vi "LEO PROVA MINCHIATA RT.vi"() -> ()   [LabVIEW 2014]
uses:
  <vilib>/FPGAPlugInAG/sbRIO-9636/niLvFpga_Open_sbRIO-9636.vi
  <vilib>/rvi/interface/common/dynamic/niFpgaDynamicAddResources.vi
  <vilib>/Utility/error.llb/Error Cluster From Error Code.vi
  <vilib>/rvi/errors/niLvFpgaAdjustHostInterfaceError.vi
  <vilib>/rvi/interface/common/niFpgaWaitOnOcc.vi
  <vilib>/FPGAPlugInAG/Dynamic/niLvFpga_Run_Dynamic.vi
  <vilib>/FPGAPlugInAG/Dynamic/niLvFpga_Abort_Dynamic.vi
  <vilib>/FPGAPlugInAG/Dynamic/niLvFpga_Close_Dynamic.vi
  <vilib>/rvi/interface/nirviOpenFPGA/nirviOpenFPGA.xnode
  FPGA Bitfiles/LaserDistanceSen_FPGATarget_LEOPROVAMINCHIAT_2r7d0oepUXA.lvbitx
  FPGA Target/Test VIs/LEO PROVA MINCHIATA.vi
  <vilib>/rvi/interface/nirviReadWriteControl/nirviReadWriteControl.xnode
  <vilib>/rvi/interface/nirviMethod/nirviMethod.xnode
  <vilib>/rvi/interface/nirviCloseFPGA/nirviCloseFPGA.xnode
  <vilib>/FPGAPlugInAG/Dynamic/niLvFpga_ConfigureFifo_Dynamic.vi
  <vilib>/rvi/errors/niLvFpgaMergeErrorWithErrorCode.vi
  <vilib>/FPGAPlugInAG/Dynamic/niLvFpga_StartFifo_Dynamic.vi
  <vilib>/rvi/interface/Simulation/niFpgaSimulationCallBeginRW.vi
  <vilib>/FPGAPlugInAG/Dynamic/niLvFpga_ReadFifo_Dynamic.vi
  NiFpgaLv.dll
panel:
  out "FFT (freq)":waveform(dbl)(graph)
  out "Signal (t)":waveform(dbl)(graph)
  in  "Snapshot":bool
  in  "Windowing":T1(ring)
  in  "first bin":i32=10
  in  "last bin":i32=255
  in  "lower limit 2":u32(slide)=677 scale=625.0..737.0
  in  "lower limit 1":u32(slide)=59 scale=0.0..112.0
  out "Detected Frequency Tone - (Hz)":dbl
  in  "stop":bool
  out "Max Bin":i32
  out "Max Amp":dbl format="%.2f"
  out "Prev Bin":i32
  out "Next Bin":i32
  out "Prev Amp":dbl format="%.2f"
  out "Next Amp":dbl format="%.2f"
  out "Interpolated Bin":dbl
  in  "Interpolation Method":T2(ring)=enum."Jain"
  # "WARNING:\nOnce pressed wait untill the end of operation"
  # "ONLINE parameter"
  # "OFFLINE parameters"
  # "Max Detection FFT bin range"
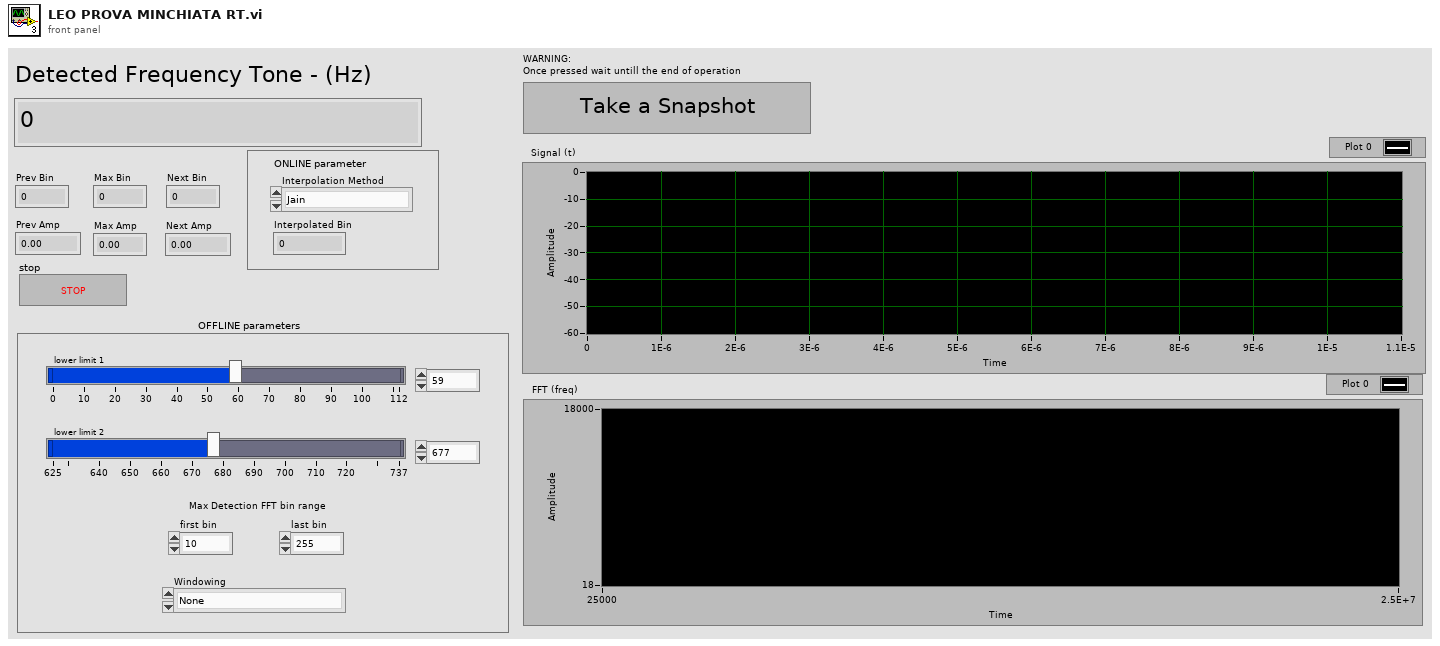
[diagram p1: front panel]
types:
  T1 = enum16{"None", "Hanning", "Hamming", "Blackman", "Blackman-Harris"}
  T2 = enum16{"Quadratic", "McLeodd", "Barycentric", "Jain"}
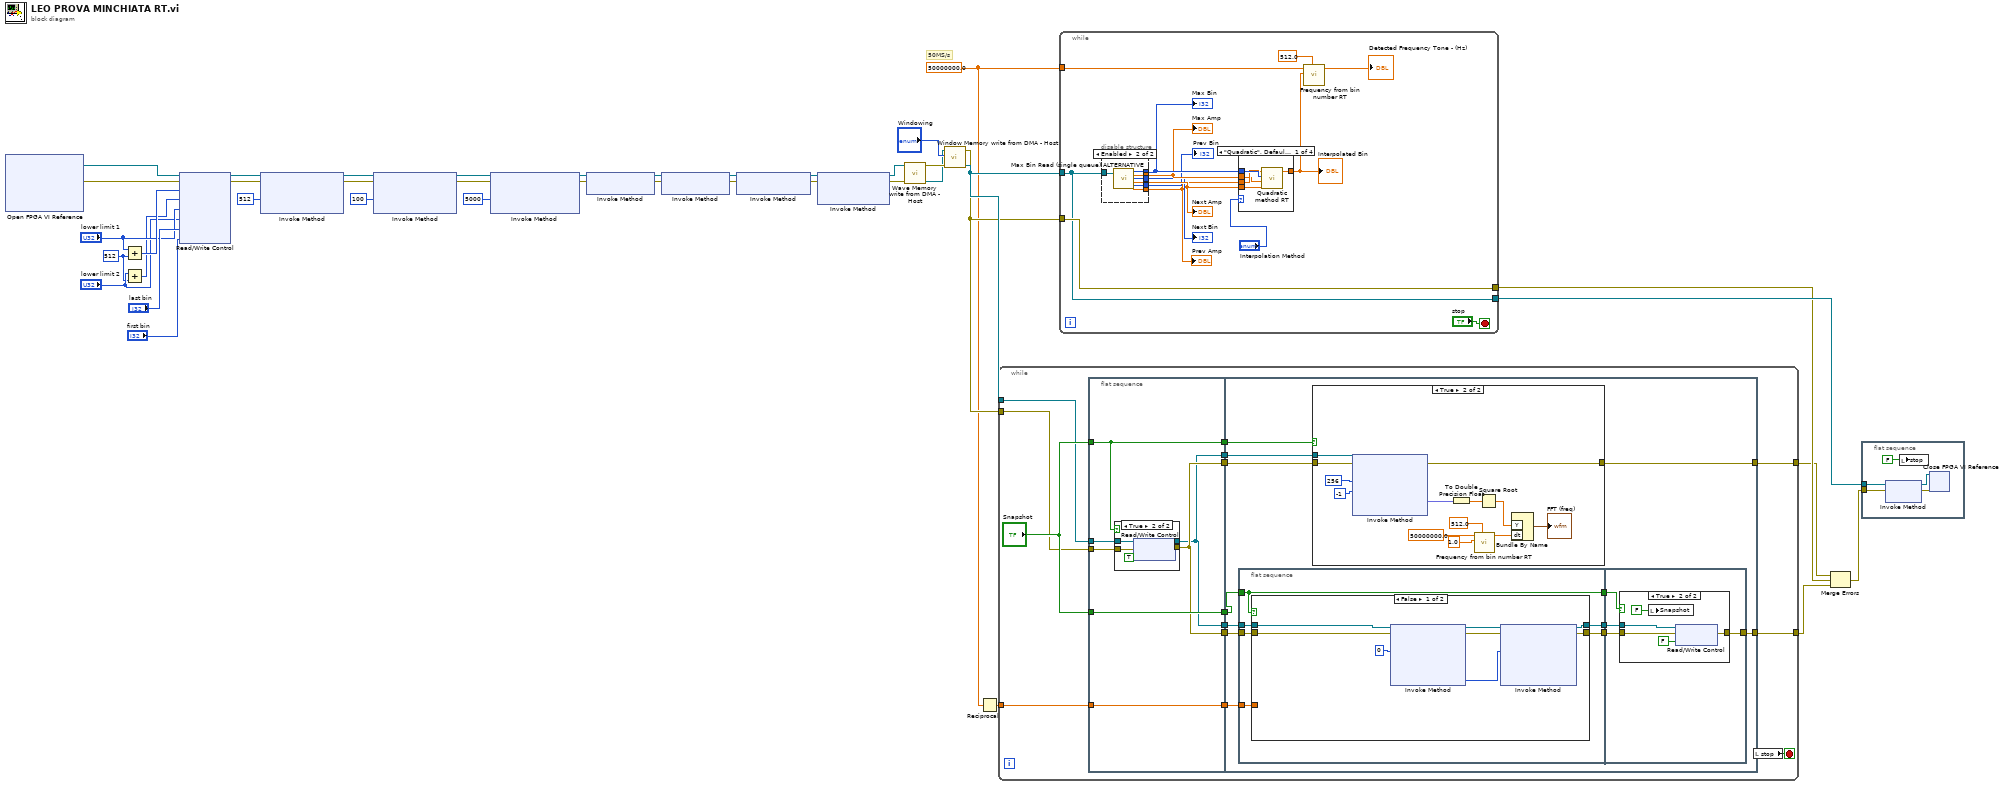
[diagram p0: block diagram]
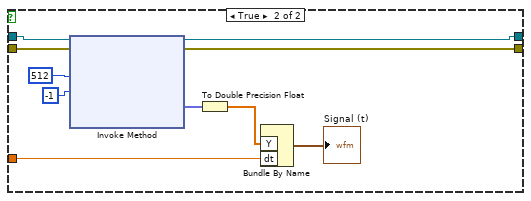
[diagram p3: hidden frame]
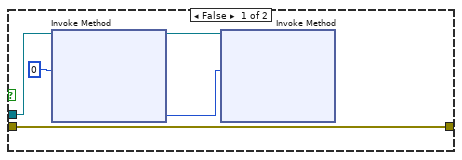
[diagram p5: hidden frame]
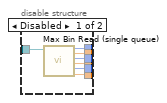
[diagram p6: hidden frame]
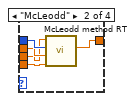
[diagram p7: hidden frame]
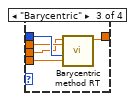
[diagram p8: hidden frame]
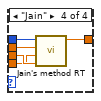
[diagram p9: hidden frame]
diagram:
  w34 = u32 512 ("y")
  w11 = 50000000.0 ("Sample Rate (S/s)")
  # "50MS/s"
  n1 = xnode "Open FPGA VI Reference"() -> ("FPGA VI Reference Out"=w33:refnum<k20>, "error out"=w32:errorcluster)  [unwired: 2 in]
  n2 = Add(x="lower limit 1", y=w34) -> (x+y=w38:u32)
  n3 = Add(x="lower limit 2", y=w34) -> (x+y=w36:u32)
  n4 = xnode "Read/Write Control"("FPGA VI Reference In"=w33, "error in"=w32, "upper limit 1"=w38, "upper limit 2"=w36, "lower limit 1"="lower limit 1", "lower limit 2"="lower limit 2", "last bin"="last bin", "first bin"="first bin") -> ("FPGA VI Reference Out"=w27:refnum<k20>, "error out"=w26:errorcluster)
  n5 = xnode "Invoke Method"("FPGA VI Reference In"=w27, "error in"=w26, "Requested Depth"=u32 512) -> ("FPGA VI Reference Out"=w25:refnum<k20>, "error out"=w24:errorcluster)  [unwired: 1 out]
  n6 = xnode "Invoke Method"("FPGA VI Reference In"=w25, "error in"=w24, "Requested Depth"=u32 100) -> ("FPGA VI Reference Out"=w23:refnum<k20>, "error out"=w22:errorcluster)  [unwired: 1 out]
  n7 = xnode "Invoke Method"("FPGA VI Reference In"=w23, "error in"=w22, "Requested Depth"=u32 5000) -> ("FPGA VI Reference Out"=w5:refnum<k20>, "error out"=w6:errorcluster)  [unwired: 1 out]
  n8 = xnode "Invoke Method"("FPGA VI Reference In"=w5, "error in"=w6) -> ("FPGA VI Reference Out"=w16:refnum<k20>, "error out"=w15:errorcluster)
  n9 = xnode "Invoke Method"("FPGA VI Reference In"=w16, "error in"=w15) -> ("FPGA VI Reference Out"=w18:refnum<k20>, "error out"=w17:errorcluster)
  n10 = xnode "Invoke Method"("FPGA VI Reference In"=w18, "error in"=w17) -> ("FPGA VI Reference Out"=w3:refnum<k20>, "error out"=w4:errorcluster)
  n11 = xnode "Invoke Method"("FPGA VI Reference In"=w3, "error in"=w4) -> ("FPGA VI Reference Out"=w10:refnum<k20>, "error out"=w9:errorcluster)  [unwired: 1 in]
  n12 = call "Wave Memory write from DMA - Host.vi"("error in"=w9, "FPGA VI Reference In"=w10) -> ("FPGA VI Reference Out"=w7:refnum<k20>, "error out"=w8:errorcluster)  [unwired: 7 in, 1 out]
  n13 = call "Window Memory write from DMA - Host.vi"("error in"=w8, "Enum"="Windowing", "FPGA VI Reference In"=w7) -> ("FPGA VI Reference Out"=w29:refnum<k20>, "error out"=w28:errorcluster)  [unwired: 5 in, 2 out]
  n14 = Reciprocal(x=w11) -> (1/x=w12:dbl)
  n15 = while {
    tunnel: w29 -> [w48]
    tunnel: w28 -> [w49]
    tunnel: [w51] -> w1
    tunnel: w12 -> [w53]
    tunnel: [w52] -> w2
    stop <- w54 stop-if-true
    n16 = flat-sequence {
      tunnel: w48 -> [w57]
      tunnel: w49 -> [w58]
      tunnel: "Snapshot" -> [w55]
      tunnel: "Snapshot" -> [w60]
      tunnel: w53 -> [w61]
      tunnel: [w59] -> w47
      tunnel: [w61] -> w46
      tunnel: [w60] -> w45
      tunnel: [w55] -> w44
      tunnel: [w59] -> w43
      tunnel: [w56] -> w42
      tunnel: [w56] -> w41
      tunnel: [w74] -> w52
      tunnel: [w72] -> w51
      tunnel: w47 -> [w76]
      tunnel: w46 -> [w75]
      tunnel: w45 -> [w73]
      tunnel: w44 -> [w71]
      tunnel: w43 -> [w70]
      tunnel: w42 -> [w69]
      tunnel: w41 -> [w77]
      frame #0 {
        n17 = case shown="True" w55 {
          tunnel: [w62 w67] -> w59
          tunnel: w58 -> [w62 w66]
          tunnel: w57 -> [w63 w65]
          tunnel: [w63 w64] -> w56
          frame False {
          }
          frame True {
            n18 = xnode "Read/Write Control"("FPGA VI Reference In"=w65, "error in"=w66, "snapshot"=TRUE) -> ("FPGA VI Reference Out"=w64:refnum<k20>, "error out"=w67:errorcluster)
          }
        }
      }
      frame #1 {
        n19 = flat-sequence {
          tunnel: w77 -> [w86]
          tunnel: w76 -> [w85]
          tunnel: w75 -> [w84]
          tunnel: w73 -> [w81]
          tunnel: [w83] -> w80
          tunnel: [w82] -> w79
          tunnel: [w81] -> w78
          tunnel: [w106] -> w72
          tunnel: w80 -> [w108]
          tunnel: w79 -> [w107]
          tunnel: w78 -> [w105]
          frame #0 {
            n20 = case shown="False" w81 {
              tunnel: w86 -> [w93 w104]
              tunnel: w85 -> [w91 w103]
              tunnel: [w90 w100] -> w82
              tunnel: w84 -> [_ w98]
              tunnel: [w87 w96] -> w83
              frame False {
                n21 = xnode "Invoke Method"("FPGA VI Reference In"=w93, "error in"=w91, "Number of Elements"=u32 0) -> ("FPGA VI Reference Out"=w89:refnum<k20>, "error out"=w88:errorcluster, "Elements Remaining"=w92:u32)  [unwired: 1 in, 1 out]
                n22 = xnode "Invoke Method"("FPGA VI Reference In"=w89, "error in"=w88, "Number of Elements"=w92) -> ("FPGA VI Reference Out"=w87:refnum<k20>, "error out"=w90:errorcluster)  [unwired: 1 in, 2 out]
              }
              frame True {
                n23 = xnode "Invoke Method"("FPGA VI Reference In"=w104, "error in"=w103, "Number of Elements"=u32 512, "Timeout (ms)"=-1) -> ("FPGA VI Reference Out"=w96:refnum<k20>, "error out"=w100:errorcluster, "Data"=w97:fxp<+/-,12,12>[])  [unwired: 1 out]
                n24 = To Double Precision Float(number=w97) -> (double precision float=w95:dbl[])
                n25 = Bundle By Name("Y"=w95, "dt"=w98) -> (→"Signal (t)":waveform(dbl))  [unwired: 1 in]
              }
            }
          }
          frame #1 {
            n26 = case shown="True" w105 {
              tunnel: [w109 w111] -> w106
              tunnel: w108 -> [_ w112]
              tunnel: w107 -> [w109 w110]
              frame False {
              }
              frame True {
                n27 = local write "Snapshot"(FALSE ("Snapshot")) -> ()
                n28 = xnode "Read/Write Control"("FPGA VI Reference In"=w112, "error in"=w110, "snapshot"=FALSE) -> ("error out"=w111:errorcluster)  [unwired: 1 out]
              }
            }
          }
        }
        n29 = case shown="True" w71 {
          tunnel: w69 -> [w117 w120]
          tunnel: w70 -> [w119 w121]
          tunnel: [w119 w132] -> w74
          frame False {
            n30 = xnode "Invoke Method"("FPGA VI Reference In"=w117, "Number of Elements"=u32 0) -> ("FPGA VI Reference Out"=w115:refnum<k20>, "Elements Remaining"=w116:u32)  [unwired: 2 in, 2 out]
            n31 = xnode "Invoke Method"("FPGA VI Reference In"=w115, "Number of Elements"=w116) -> ()  [unwired: 2 in, 4 out]
          }
          frame True {
            n32 = xnode "Invoke Method"("FPGA VI Reference In"=w120, "error in"=w121, "Number of Elements"=u32 256, "Timeout (ms)"=-1) -> ("error out"=w132:errorcluster, "Data"=w129:fxp<+,44,44>[])  [unwired: 2 out]
            n33 = To Double Precision Float(number=w129) -> (double precision float=w128:dbl[])
            n34 = call "Frequency from bin number RT.vi"("FFT size"=512.0, "Bin number"=1.0, "Sample Rate (S/s)"=50000000.0) -> ("Detected Frequency (Hz)"=w124:dbl)  [unwired: 8 in]
            n35 = Square Root(x=w128) -> (sqrt(x)=w123:dbl[])
            n36 = Bundle By Name("Y"=w123, "dt"=w124) -> (→"FFT (freq)":waveform(dbl))  [unwired: 1 in]
          }
        }
      }
    }
    n37 = local read "stop"() -> (w54:bool)
  }
  n38 = while {
    tunnel: w11 -> [w145]
    tunnel: w29 -> [w143]
    tunnel: w28 -> [w144]
    tunnel: [w143] -> w31
    tunnel: [w144] -> w14
    stop <- "stop" stop-if-true
    n39 = disable-structure shown="Enabled" {
      disable-tunnel: w143 -> [w153 w160]
      disable-tunnel: [w152 w159] -> w139
      disable-tunnel: [w151 w158] -> w138
      disable-tunnel: [w150 w156] -> w137
      disable-tunnel: [w149 w154] -> w136
      disable-tunnel: [w148 w155] -> w135
      disable-tunnel: [w147 w157] -> w134
      frame Disabled {
        n40 = call "Max Bin Read (single queue).vi"("FPGA VI Reference In"=w153) -> ("Max Bin"=w152:i32, "Max Amp"=w151:dbl, "Next Bin"=w147:i32, "Next Amp"=w150:dbl, "Prev Bin"=w148:i32, "Prev Amp"=w149:dbl)  [unwired: 13 in]
      }
      frame Enabled {
        n41 = call "Max Bin Read (single queue) ALTERNATIVE.vi"("FPGA VI Reference In"=w160) -> ("Max Bin"=w159:i32, "Max Amp"=w158:dbl, "Next Bin"=w157:i32, "Next Amp"=w156:dbl, "Prev Bin"=w155:i32, "Prev Amp"=w154:dbl)  [unwired: 13 in]
      }
    }
    "Max Bin" <- w139
    "Max Amp" <- w138
    "Prev Bin" <- w135
    "Next Bin" <- w134
    "Prev Amp" <- w136
    "Next Amp" <- w137
    n42 = case shown="\"Quadratic\", Default" "Interpolation Method" {
      tunnel: w139 -> [w164 w169 w174 w179]
      tunnel: w138 -> [w161 w168 w173 w178]
      tunnel: w136 -> [w162 w167 w172 w177]
      tunnel: w137 -> [w163 w166 w171 w176]
      tunnel: [w165 w170 w175 w180] -> w140
      frame "Quadratic", Default {
        n43 = call "Quadratic method RT.vi"("Next Amplitude"=w163, "Max Amplitude"=w161, "Max bin"=w164, "Prev Amplitude"=w162) -> ("Bin"=w165:dbl)  [unwired: 7 in]
      }
      frame "McLeodd" {
        n44 = call "McLeodd method RT.vi"("Next Amp"=w166, "Max Amp"=w168, "Max Bin"=w169, "Prev Amp"=w167) -> ("Bin"=w170:dbl)  [unwired: 7 in]
      }
      frame "Barycentric" {
        n45 = call "Barycentric method RT.vi"("Next Amp"=w171, "Max Bin"=w174, "Max Amp"=w173, "Prev Amp"=w172) -> ("Bin"=w175:dbl)  [unwired: 7 in]
      }
      frame "Jain" {
        n46 = call "Jain's method RT.vi"("Prev Amp"=w177, "Next Amp"=w176, "Max Amp"=w178, "Max Bin"=w179) -> ("Bin"=w180:dbl)  [unwired: 7 in]
      }
    }
    "Interpolated Bin" <- w140
    n47 = call "Frequency from bin number RT.vi"("FFT size"=512.0, "Bin number"=w140, "Sample Rate (S/s)"=w145) -> ("Detected Frequency (Hz)"=→"Detected Frequency Tone - (Hz)":dbl)  [unwired: 8 in]
  }
  n48 = Merge Errors(w2, w14, w1) -> (w13:errorcluster)
  n49 = flat-sequence {
    tunnel: w31 -> [w183]
    tunnel: w13 -> [w182]
    frame #0 {
      n50 = xnode "Invoke Method"("FPGA VI Reference In"=w183, "error in"=w182) -> ("FPGA VI Reference Out"=w184:refnum<k20>, "error out"=w185:errorcluster)
      n51 = local write "stop"(FALSE ("stop")) -> ()
      n52 = xnode "Close FPGA VI Reference"("FPGA VI Reference In"=w184, "error in"=w185) -> ()  [unwired: 1 out]
    }
  }
